vi "Mobility-Vt Calculator_Linear.vi"(0 "Vg Column":dbl[](array[numeric]), 1 "Vd":dbl, 5 "Lin Id Column":dbl[](array[numeric]), 7 "NumPts":i32=5, 9 "Length":dbl, 11 "Width":dbl, 12 "Dielectric Thickness":dbl, 13 "Dielectric Constant":dbl) -> (2 "Used Points":cluster{"Vg Used":dbl[], "Sqrt(Id) Used ":dbl[]}, 3 "Lin Log":cluster{dbl[], dbl[]}[](graph), 4 "Mobility-Lin":dbl format="%#_4e", 6 "VT-Lin":dbl, 8 "Index-Lin":dbl, 10 "Lin Plot":cluster{dbl[], dbl[]}[](graph), 14 "Raw Graph":cluster{dbl[], dbl[]}[](graph))   [LabVIEW 2012]
uses:
  <vilib>/Analysis/NI_AALPro.lvlib
panel:
  out "Capacitance (C)":dbl
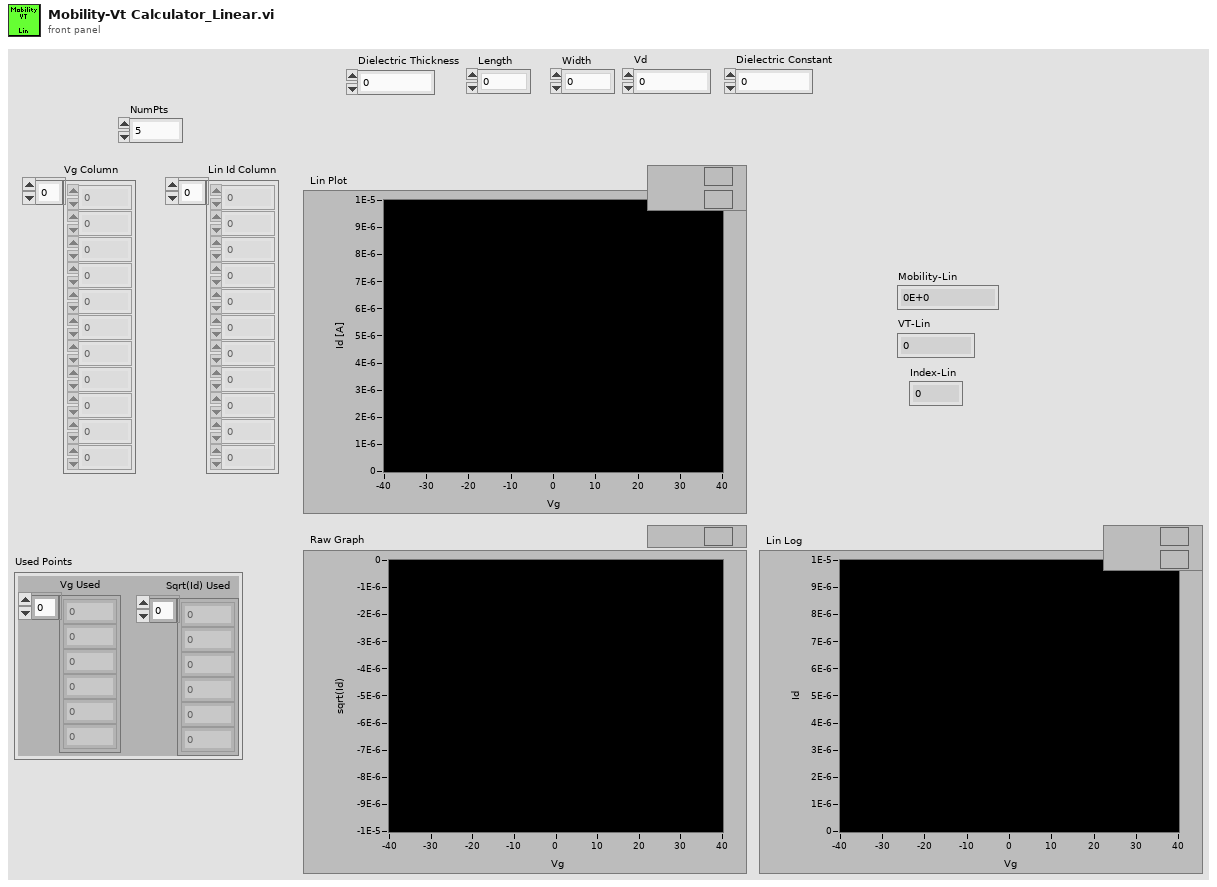
[diagram p1: front panel]
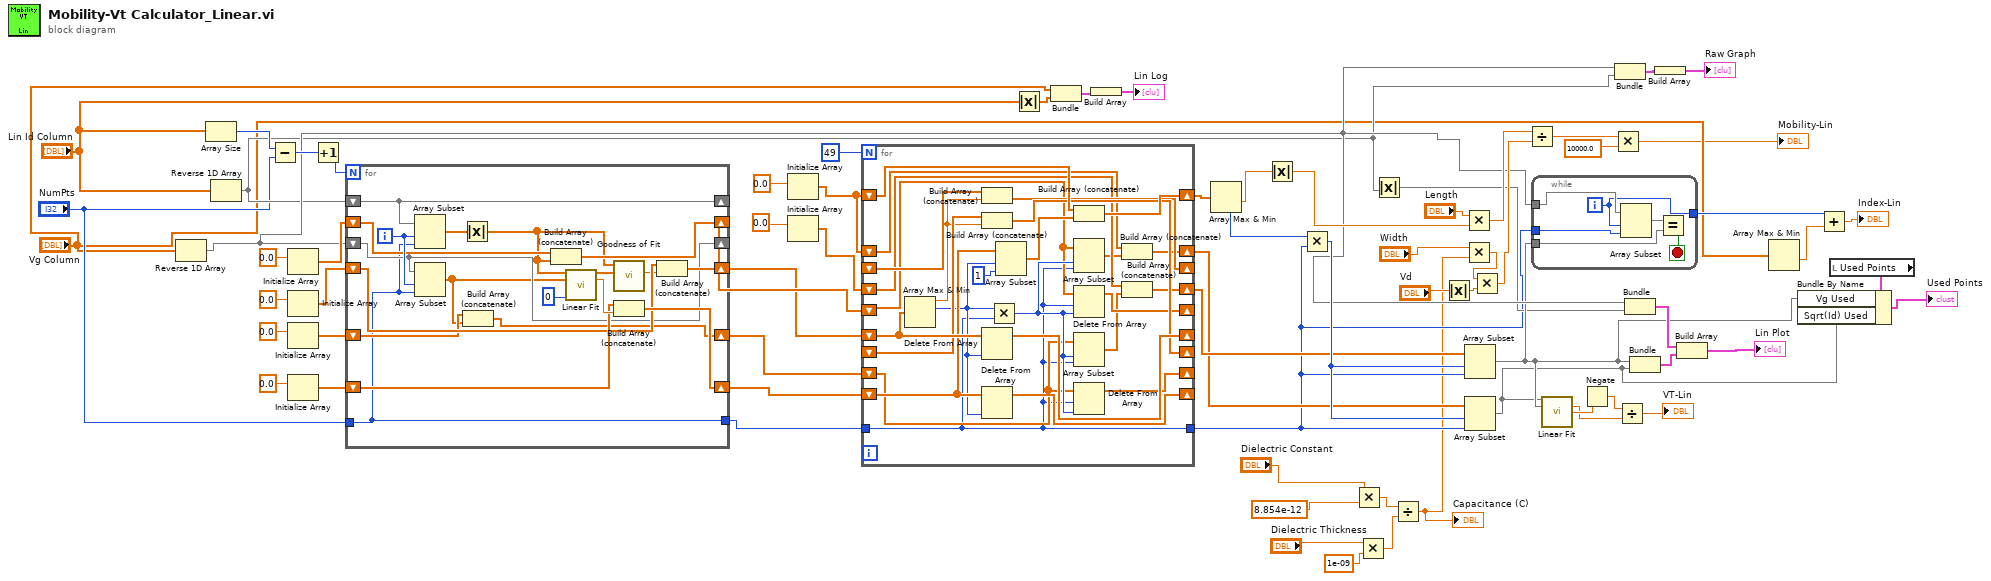
[diagram p0: block diagram]
diagram:
  n1 = Reverse 1D Array(array="Vg Column") -> (reversed array=w26:dbl[])
  n2 = Array Size(array="Lin Id Column") -> (size(s)=w38:i32)
  n3 = Reverse 1D Array(array="Lin Id Column") -> (reversed array=w25:dbl[])
  n4 = Subtract(x=w38, y="NumPts") -> (x-y=w69:i32)
  n5 = Initialize Array(0.0) -> (w57:dbl[])  [unwired: 1 in]
  n6 = Initialize Array(0.0) -> (w47:dbl[])  [unwired: 1 in]
  n7 = Initialize Array(0.0) -> (w58:dbl[])  [unwired: 1 in]
  n8 = Initialize Array(0.0) -> (w46:dbl[])  [unwired: 1 in]
  n9 = Increment(x=w69) -> (x+1=w70:i32)
  n10 = for {
    N: w70 -> [_]
    shift-right: [w77] -> _
    shift-left: w26 -> [w77]
    shift-right: [w84] -> _
    shift-left: w25 -> [w84]
    shift-right: [w88] -> w51
    shift-left: w46 -> [w87]
    shift-right: [w86] -> w53
    shift-left: w47 -> [w85]
    tunnel: "NumPts" -> [w72]
    shift-right: [w80] -> w59
    shift-left: w57 -> [w81]
    shift-right: [w78] -> w60
    shift-left: w58 -> [w79]
    tunnel: [w72] -> w12
    i -> [w90]
    n11 = Array Subset(array=w84, index=w90, length=w72) -> (w83:dbl[])
    n12 = Array Subset(array=w77, index=w90, length=w72) -> (w76:dbl[])
    n13 = Absolute Value(x=w83) -> (abs(x)=w73:dbl[])
    n14 = Build Array (concatenate)(w79, w76) -> (w78:dbl[])
    n15 = Build Array (concatenate)(w81, w73) -> (w80:dbl[])
    n16 = call <vilib>:"Linear Fit.vi"("Y"=w73, "X"=w76, "method"=0) -> ("Best Linear Fit"=w75:dbl[], "slope"=w89:dbl)  [unwired: 8 in, 3 out]
    n17 = call <vilib>:"Goodness of Fit.vi"("Best Fit"=w75, "Y"=w73) -> ("R-square"=w74:dbl)  [unwired: 6 in, 3 out]
    n18 = Build Array (concatenate)(w87, w89) -> (w88:dbl[])
    n19 = Build Array (concatenate)(w85, w74) -> (w86:dbl[])
  }
  n20 = Initialize Array(0.0) -> (w66:dbl[])  [unwired: 1 in]
  n21 = Initialize Array(0.0) -> (w61:dbl[])  [unwired: 1 in]
  n22 = for {
    N: 49 -> [_]
    shift-right: [w115] -> _
    shift-left: w53 -> [w116]
    shift-right: [w96] -> _
    shift-left: w51 -> [w97]
    shift-right: [w112] -> w52
    shift-left: w66 -> [w111]
    shift-right: [w110] -> _
    shift-left: _ -> [w109]
    shift-right: [w108] -> _
    shift-left: _ -> [w107]
    shift-right: [w106] -> _
    shift-left: w59 -> [w93]
    shift-right: [w104] -> _
    shift-left: w60 -> [w92]
    tunnel: w12 -> [w91]
    shift-right: [w103] -> w63
    shift-left: w66 -> [w102]
    shift-right: [w101] -> w64
    shift-left: w61 -> [w100]
    tunnel: [w91] -> w11
    n23 = Array Max & Min(array=w116) -> (max value=w95:dbl, max index (indices)=w94:i32)  [unwired: 2 out]
    n24 = Build Array (concatenate)(w107, w95) -> (w108:dbl[])
    n25 = Build Array (concatenate)(w109, w95) -> (w110:dbl[])
    n26 = Delete From Array(array=w116, index=w94) -> (array with subset deleted=w115:dbl[])  [unwired: 1 in, 1 out]
    n27 = Delete From Array(array=w97, index=w94) -> (array with subset deleted=w96:dbl[])  [unwired: 1 in, 1 out]
    n28 = Multiply(x=w94, y=w91) -> (x*y=w105:i32)
    n29 = Array Subset(array=w97, index=w94, length=1) -> (w113:dbl[])
    n30 = Build Array (concatenate)(w111, w113) -> (w112:dbl[])
    n31 = Array Subset(array=w93, index=w105, length=w91) -> (w98:dbl[])
    n32 = Delete From Array(array=w93, length=w91, index=w105) -> (array with subset deleted=w106:dbl[])  [unwired: 1 out]
    n33 = Array Subset(array=w92, index=w105, length=w91) -> (w99:dbl[])
    n34 = Delete From Array(array=w92, length=w91, index=w105) -> (array with subset deleted=w104:dbl[])  [unwired: 1 out]
    n35 = Build Array (concatenate)(w102, w98) -> (w103:dbl[])
    n36 = Build Array (concatenate)(w100, w99) -> (w101:dbl[])
  }
  n37 = Absolute Value(x="Lin Id Column") -> (abs(x)=w22:dbl[])
  n38 = Bundle("Vg Column"="Vg Column", w22) -> (w24:cluster{"Vg Column":dbl[], dbl[]})  [unwired: 1 in]
  n39 = Build Array(w24) -> (→"Lin Log":cluster{"Vg Column":dbl[], dbl[]}[])
  n40 = Array Max & Min(array=w52) -> (min value=w31:dbl, min index (indices)=w65:i32)  [unwired: 2 out]
  n41 = Absolute Value(x=w31) -> (abs(x)=w30:dbl)
  n42 = Multiply(x=w65, y=w11) -> (x*y=w67:i32)
  n43 = Multiply(x="Dielectric Constant", y=8.854e-12) -> (x*y=w35:dbl)
  n44 = Multiply(x="Dielectric Thickness", y=1e-09) -> (x*y=w33:dbl)
  n45 = Absolute Value(x=w25) -> (abs(x)=w14:dbl[])
  n46 = Divide(x=w35, y=w33) -> (x/y=w3:dbl)
  "Capacitance (C)" <- w3
  n47 = Absolute Value(x="Vd") -> (abs(x)=w29:dbl)
  n48 = Multiply(x="Length", y=w30) -> (x*y=w45:dbl)
  n49 = Multiply(x="Width", y=w3) -> (x*y=w36:dbl)
  n50 = Array Subset(array=w64, index=w67, length=w11) -> (w16:dbl[])
  n51 = Array Subset(array=w63, index=w67, length=w11) -> (w15:dbl[])
  n52 = Multiply(x=w36, y=w29) -> (x*y=w37:dbl)
  n53 = Divide(x=w45, y=w37) -> (x/y=w44:dbl)
  n54 = while {
    tunnel: w26 -> [w121]
    tunnel: w16 -> [w120]
    tunnel: [w118] -> w21
    tunnel: w11 -> [w117]
    i -> [w118]
    stop <- w122 stop-if-true
    n55 = Array Subset(array=w121, index=w118, length=w117) -> (w119:dbl[])
    n56 = Equal?(x=w119, y=w120) -> (x = y?=w122:bool)
  }
  n57 = call <vilib>:"Linear Fit.vi"("Y"=w15, "X"=w16) -> ("slope"=w40:dbl, "intercept"=w42:dbl)  [unwired: 9 in, 3 out]
  n58 = Negate(x=w42) -> (-x=w41:dbl)
  n59 = Multiply(x=w44, y=10000.0) -> (x*y=→"Mobility-Lin":dbl)
  n60 = Bundle(w26, w25) -> (w27:cluster{dbl[], dbl[]})  [unwired: 1 in]
  n61 = Divide(x=w41, y=w40) -> (x/y=→"VT-Lin":dbl)
  n62 = Bundle(w26, w14) -> (w55:cluster{dbl[], dbl[]})  [unwired: 1 in]
  n63 = Bundle(w16, w15) -> (w68:cluster{dbl[], dbl[]})  [unwired: 1 in]
  n64 = Build Array(w27) -> (→"Raw Graph":cluster{dbl[], dbl[]}[])
  n65 = Build Array(w55, w68) -> (→"Lin Plot":cluster{dbl[], dbl[]}[])
  n66 = Array Max & Min(array="Vg Column") -> (min value=w20:dbl)  [unwired: 3 out]
  n67 = Add(x=w21, y=w20) -> (x+y=→"Index-Lin":dbl)
  n68 = local read "Used Points"() -> (w17:cluster{"Vg Used":dbl[], "Sqrt(Id) Used ":dbl[]})
  n69 = Bundle By Name(cluster=w17, "Vg Used"=w16, "Sqrt(Id) Used"=w15) -> (→"Used Points":cluster{"Vg Used":dbl[], "Sqrt(Id) Used ":dbl[]})
